vi "GFITS_openImage.lv12.vi"() -> ()   [LabVIEW 2012]
uses:
  c/lib/libgfits.so
panel:
  out "err 2":i32
  in  "err":i32
  in  "imname":string="/home/bonati/images/chiron/test.fits"
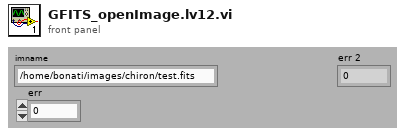
[diagram p1: front panel]
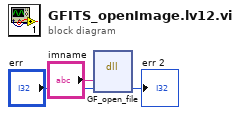
[diagram p0: block diagram]
diagram:
  n1 = dll-call lib="home/bonati/panview_current/PAN/Modules/GFITS.lv86/private/c/lib/libgfits.so" fn="GF_open_file"("imname"="imname", "err"="err") -> ("err"=→"err 2":i32)  [unwired: 3 in, 4 out]
